vi "Prepare Logger.vi"(8 "error in (no error)":errorcluster, 10 "Prepare Log":T1, 11 "MsgQ in":refnum<class "MessageQ.lvclass">) -> (0 "error out":errorcluster, 3 "MsgQ":refnum<class "MessageQ.lvclass">)   [LabVIEW 2020, in "VolatusData.lvlib"]
uses:
  VolatusData.lvlib
  Volatus/MessageQ/MessageQ.lvclass
  Prepare Log.ctl
  Volatus/MessageQ/MessageQ.lvclass/MessageQ.ctl
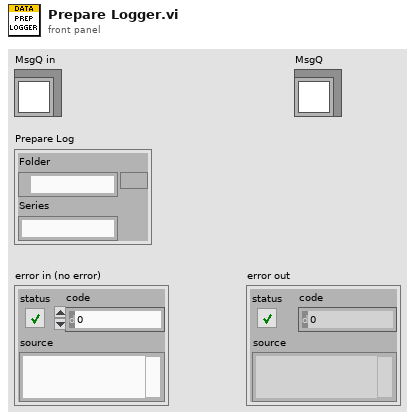
[diagram p1: front panel]
types:
  T1 = typedef "VolatusData.lvlib/Prepare Log.ctl" = cluster{"Folder":path, "Series":string}
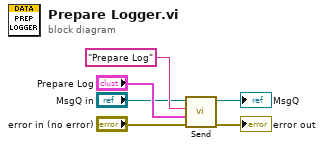
[diagram p0: block diagram]
diagram:
  n1 = call "Send.vi"("error in (no error)"="error in (no error)", "Data"="Prepare Log", "ID"="Prepare Log", "MessageQ in"="MsgQ in") -> ("error out"=→"error out":errorcluster, "MessageQ out"=→"MsgQ":refnum<class "MessageQ.lvclass">)  [unwired: 6 in]
